vi "RT Driver VI.vi"(7 "Operation":T1, 11 "Device Reference in":T2 format="%.0x") -> (0 "Error Code":i32)   [LabVIEW 2017, in "Data Sharing Framework Engine.lvlib"]
uses:
  Data Sharing Framework Engine.lvlib
  <vilib>/NI Veristand/Custom Device API/Custom Device Item Ref.ctl
  <vilib>/NI Veristand/Custom Device API/Hardware Interface Driver VI Operation.ctl
  VeriStand Framework/VeriStand Data Sharing Framework.lvclass
  DSF Core.lvlibp/Classes/Framework/Framework Options.ctl
  DSF Core.lvlibp/Typedefs/DSF FIFO Options.ctl
  DSF Core.lvlibp/Classes/Thread/DSF Thread Options.ctl
  DSF Core.lvlibp/Typedefs/DSF Plugin Options.ctl
  DSF Core.lvlibp/Typedefs/DSF Performance Options.ctl
  <vilib>/NI Veristand/Custom Device API/Global Data Refs.vi
  DSF Core.lvlibp/Classes/Framework/Set Framework Cycle.vi
  DSF Core.lvlibp/Classes/Framework/Active Plugins.vi
  DSF Core.lvlibp/Classes/Framework/Receive.vi
  <vilib>/NI Veristand/Custom Device API/Custom Device API.lvlib
  DSF Core.lvlibp/Classes/Framework/Framework.lvclass
  DSF Core.lvlibp
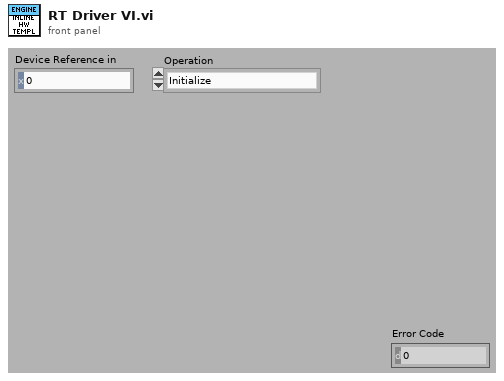
[diagram p1: front panel]
types:
  T1 = typedef "Custom Device API.lvlib/Hardware Interface Driver VI Operation.ctl" = enum16{"Initialize", "Start", "Read Data from HW", "Write Data to HW", "Close"}
  T2 = typedef "Custom Device API.lvlib/Custom Device Item Ref.ctl" = u64
  T3 = typedef "DSF Core.lvlibp/Framework.lvclass/Framework Options.ctl" = cluster{"FIFO Options":T4, "Thread Options":T5, "Plugin Options":T6, "Performance Options":T7}
  T4 = typedef "DSF Core.lvlibp/DSF FIFO Options.ctl" = cluster{"Infinite Timeouts":bool}
  T5 = typedef "DSF Core.lvlibp/DSF Thread Options.ctl" = cluster{"Show FP On Call":bool, "Close FP After Call":bool, "Allow Debugging":bool, "Show Menu Bar":bool, "Reposition Windows":bool}
  T6 = typedef "DSF Core.lvlibp/DSF Plugin Options.ctl" = cluster{"Default Components":bool}
  T7 = typedef "DSF Core.lvlibp/DSF Performance Options.ctl" = cluster{"Measure Period":bool, "Measure Rx/Tx Duration":bool}
  T8 = typedef "Custom Device API.lvlib/Data Table Ref.ctl" = cluster{"Ptr.Beg":u64, "Ptr.End":u64}
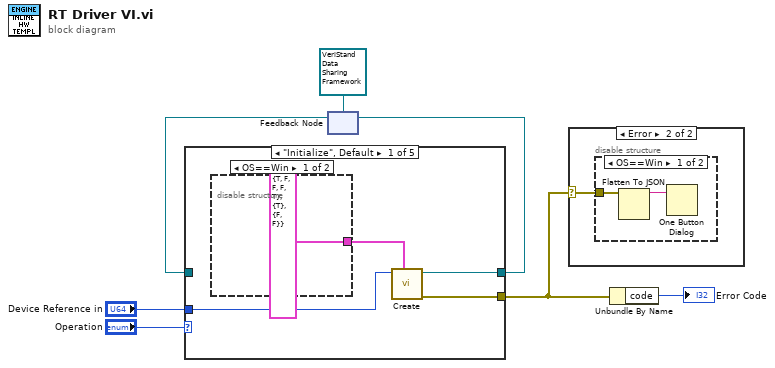
[diagram p0: block diagram]
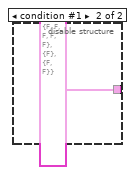
[diagram p4: hidden frame]
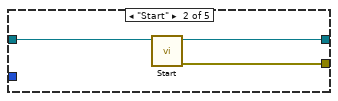
[diagram p5: hidden frame]
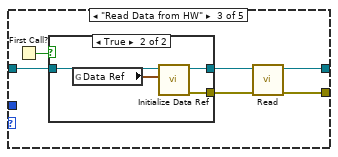
[diagram p6: hidden frame]
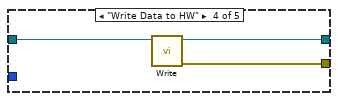
[diagram p8: hidden frame]
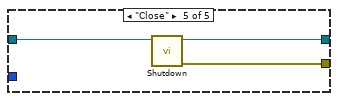
[diagram p9: hidden frame]
diagram:
  n1 = feedback #1(refnum<class "VeriStand Data Sharing Framework.lvclass"> refnum ("Data Sharing Framework Engine.lvlib:VeriStand Data Sharing Framework.lvclass")) -> (w7:refnum<class "VeriStand Data Sharing Framework.lvclass">)
  n2 = case shown="\"Initialize\", Default" "Operation" {
    tunnel: [w8 w15 w20 w29 w31] -> w5
    tunnel: w7 -> [_ w16 w21 w30 w33]
    tunnel: "Device Reference in" -> [w10 _ _ _ _]
    tunnel: [w11 w14 w17 w28 w32] -> w1
    frame "Initialize", Default {
      n3 = disable-structure shown="OS==Win" {
        disable-tunnel: [T3 {"FIFO Options"={"Infinite Timeouts"=TRUE}, "Thread Options"={"Show FP On Call"=TRUE, "Close FP After Call"=FALSE, "Allow Debugging"=FALSE, "Show Menu Bar"=FALSE, "Reposition Windows"=TRUE}, "Plugin Options"={"Default Components"=TRUE}, "Performance Options"={"Measure Period"=FALSE, "Measure Rx/Tx Duration"=FALSE}} ("options") T3 {"FIFO Options"={"Infinite Timeouts"=FALSE}, "Thread Options"={"Show FP On Call"=FALSE, "Close FP After Call"=FALSE, "Allow Debugging"=FALSE, "Show Menu Bar"=FALSE, "Reposition Windows"=FALSE}, "Plugin Options"={"Default Components"=FALSE}, "Performance Options"={"Measure Period"=FALSE, "Measure Rx/Tx Duration"=FALSE}} ("options")] -> w9
        frame condition #0 (active) {
        }
        frame condition #1 {
        }
      }
      n4 = call "Create.vi"("options"=w9, "Device Item Ref"=w10) -> ("error out"=w11:errorcluster, "VeriStand Framework"=w8:refnum<class "VeriStand Data Sharing Framework.lvclass">)  [unwired: 8 in]
    }
    frame "Start" {
      n5 = call-dynamic "Start.vi"("VeriStand Data Sharing Framework in"=w16) -> ("error out"=w14:errorcluster, "VeriStand Data Sharing Framework out"=w15:refnum<class "VeriStand Data Sharing Framework.lvclass">)  [unwired: 9 in]
    }
    frame "Read Data from HW" {
      n6 = First Call?() -> (First Call?: T/F=w22:bool)
      n7 = case shown="True" w22 {
        tunnel: w21 -> [w23 w27]
        tunnel: [w23 w26] -> w19
        tunnel: [_ w25] -> w18
        frame False {
        }
        frame True {
          n8 = global read "Global Data Refs.vi" "Data Ref"() -> (w24:T8)
          n9 = call "Initialize Data Ref.vi"("Data Ref"=w24, "VeriStand Data Sharing Framework in"=w27) -> ("error out"=w25:errorcluster, "VeriStand Data Sharing Framework out"=w26:refnum<class "VeriStand Data Sharing Framework.lvclass">)  [unwired: 8 in]
        }
      }
      n10 = call "Read.vi"("error in (no error)"=w18, "VeriStand DSF in"=w19) -> ("error out"=w17:errorcluster, "VeriStand DSF out"=w20:refnum<class "VeriStand Data Sharing Framework.lvclass">)  [unwired: 8 in]
    }
    frame "Write Data to HW" {
      n11 = call "Write.vi"("VeriStand Data Sharing Framework in"=w30) -> ("error out"=w28:errorcluster, "VeriStand Data Sharing Framework out"=w29:refnum<class "VeriStand Data Sharing Framework.lvclass">)  [unwired: 9 in]
    }
    frame "Close" {
      n12 = call-dynamic "Shutdown.vi"("VeriStand Data Sharing Framework in"=w33) -> ("error out"=w32:errorcluster, "VeriStand Data Sharing Framework out"=w31:refnum<class "VeriStand Data Sharing Framework.lvclass">)  [unwired: 9 in]
    }
  }
  n13 = feedback-in #1(w5) -> ()
  n14 = case shown="Error" w1 {
    selector: w1 -> [_ w34]
    frame No Error {
    }
    frame Error {
      n15 = disable-structure shown="OS==Win" {
        disable-tunnel: w34 -> [w36 _]
        frame condition #0 (active) {
          n16 = Flatten To JSON(anything=w36) -> (JSON string=w35:string)  [unwired: 2 in, 1 out]
          n17 = One Button Dialog(message=w35) -> ()  [unwired: 1 in, 1 out]
        }
        frame condition #1 {
        }
      }
    }
  }
  n18 = Unbundle By Name(w1) -> ("code"=→"Error Code":i32)
